vi "纳清pH_所有参数读取.vi"(8 "error in (no error)":errorcluster caption="错误输入（无错误）", 11 "MB session in":refnum<class "MB_Master.lvclass">) -> (0 "error out":errorcluster caption="错误输出", 2 "输出值":T1 {"波特率" items=["4800", "9600", "19200", "38400", "57600", "115200"]}, 3 "MB session out":refnum<class "MB_Master.lvclass">)   [LabVIEW 2016, in "斯坦道多参数.lvlib"]
uses:
  <vilib>/Plasmionique/MB Master/MB_Master/MB_Master.lvclass
  <vilib>/Plasmionique/MB Master/MB Master.lvlib
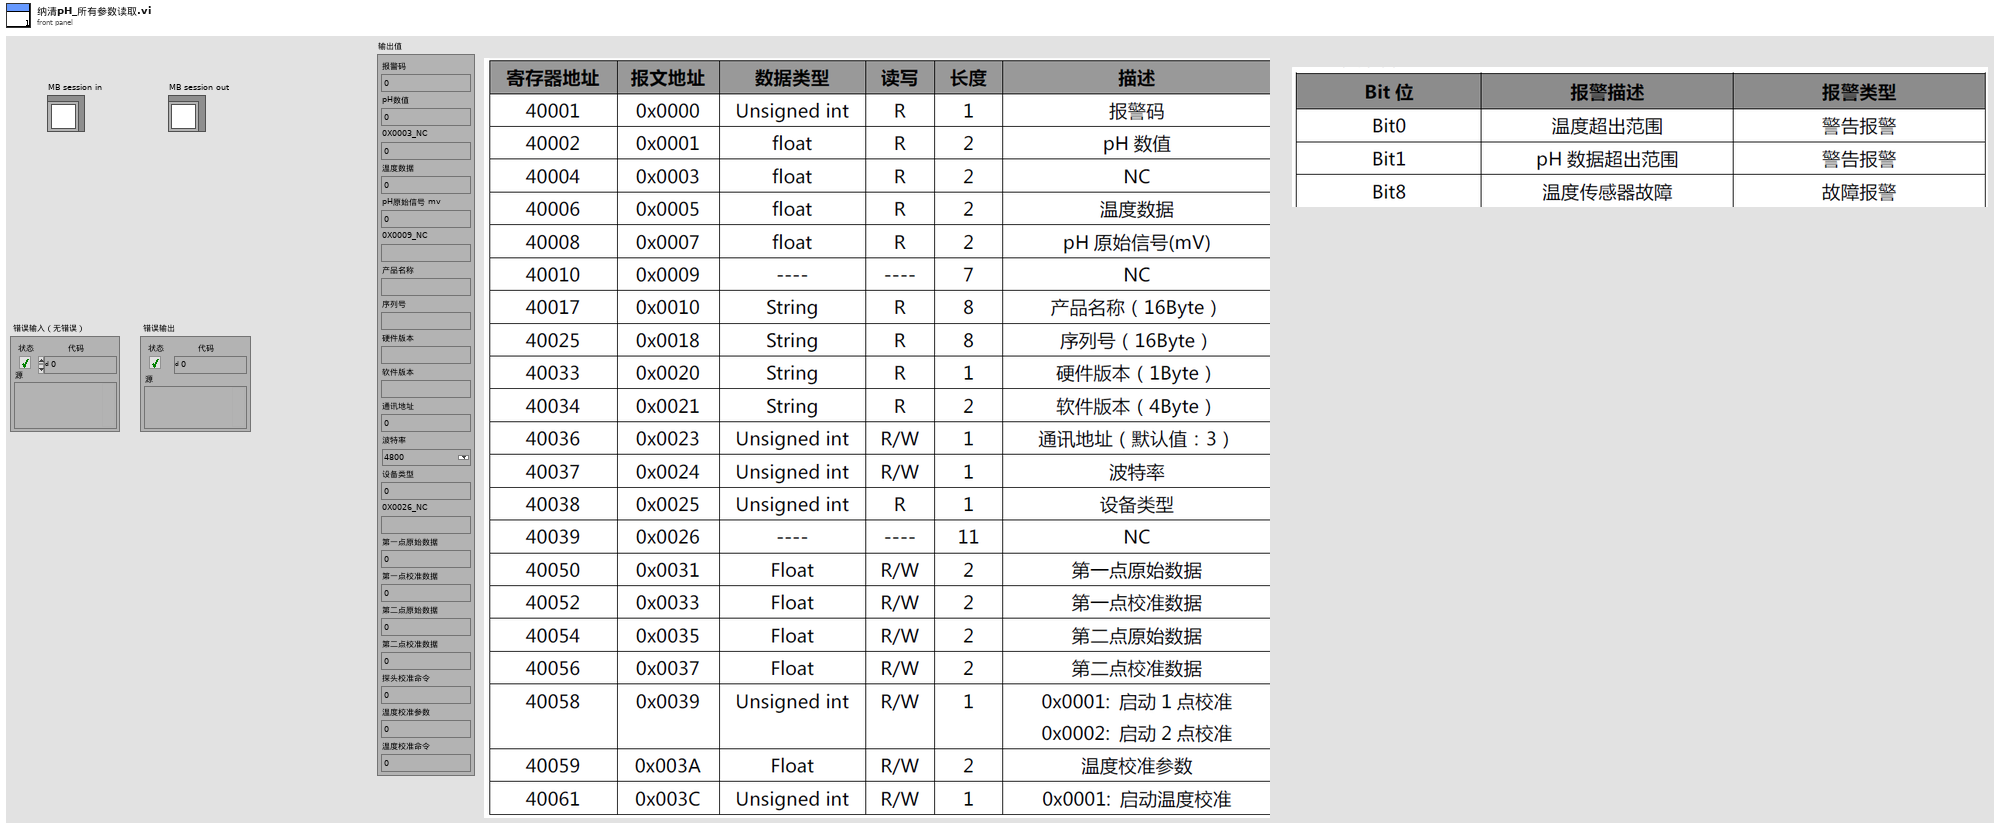
[diagram p1: front panel]
types:
  T1 = cluster{"报警码":u16, "pH数值":sgl, "0X0003_NC":sgl, "温度数据":sgl, "pH原始信号 mv":sgl, "0X0009_NC":string, "产品名称":string, "序列号":string, "硬件版本":string, "软件版本":string, "通讯地址":u16, "波特率":u16, "设备类型":u16, "0X0026_NC":string, "第一点原始数据":sgl, "第一点校准数据":sgl, "第二点原始数据":sgl, "第二点校准数据":sgl, "探头校准命令":u16, "温度校准参数":sgl, "温度校准命令":u16}
  T2 = cluster{"pH":u32, "DO":u32, "Cond":u32, "Turb":u32, "叶绿素a":u32, "藻密度":u32, "ORP":u32}
  T3 = cluster{u16, "mode":dbl, "数值":sgl, "数值":sgl, "数值":sgl, "类型":string, "类型":string, "类型":string, "类型":string, "类型":string, u16, u16, u16, "类型":string, "数值":sgl, "数值":sgl, "数值":sgl, "数值":sgl, u16, "数值":sgl, u16}
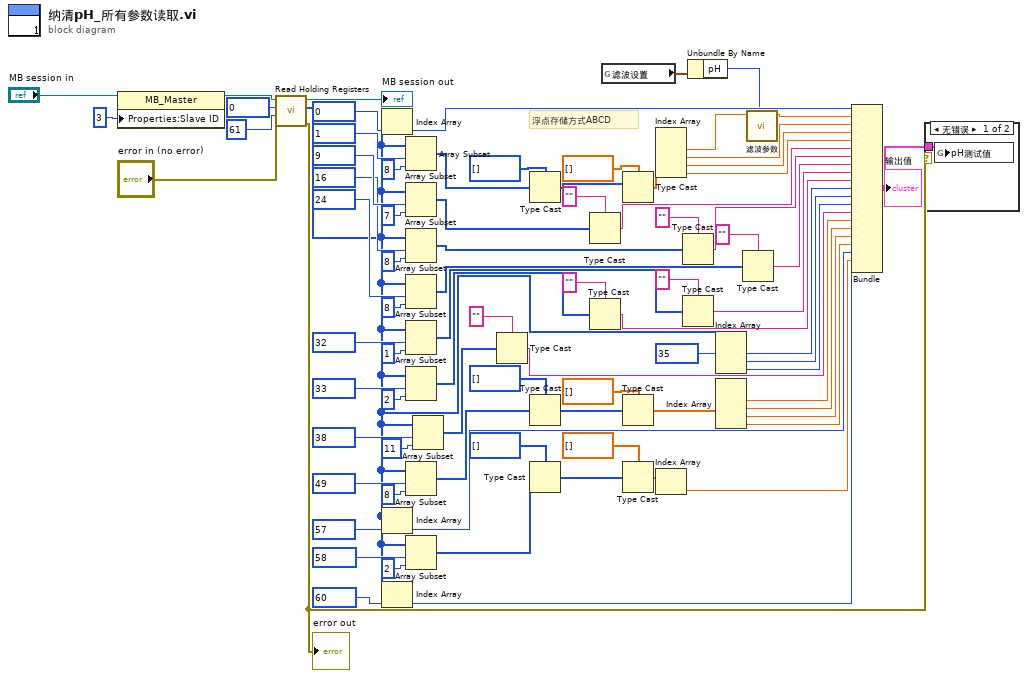
[diagram p0: block diagram]
diagram:
  # "浮点存储方式ABCD"
  n1 = property class="MB_Master"(reference="MB session in", "Properties:Slave ID"=u8 3 ("Slave ID")) -> (reference out=w73:refnum<class "MB_Master.lvclass">)  [unwired: 1 in, 1 out]
  n2 = call <vilib>:"Read Holding Registers.vi"("error in (no error)"="error in (no error)", "quantity"=u16 61, "starting address"=u16 0, "MB session in"=w73) -> ("error out"=w14:errorcluster, "Registers"=w16:u16[], "MB session out"=→"MB session out":refnum<class "MB_Master.lvclass">)  [unwired: 5 in]
  "error out" <- w14
  n3 = Index Array(array=w16, index=u16 0 ("starting address")) -> (element=w81:u16)
  n4 = Index Array(array=w16, index=u16 57 ("starting address")) -> (element=w19:u16)
  n5 = Index Array(array=w16, index=u16 60 ("starting address")) -> (element=w15:u16)
  n6 = Array Subset(array=w16, index=u16 1 ("starting address"), length=8 ("长度")) -> (w77:u16[])
  n7 = Array Subset(array=w16, index=u16 9 ("starting address"), length=7 ("长度")) -> (w67:u16[])
  n8 = Array Subset(array=w16, index=u16 16 ("starting address"), length=8 ("长度")) -> (w63:u16[])
  n9 = Array Subset(array=w16, index=u16 24 ("starting address"), length=8 ("长度")) -> (w57:u16[])
  n10 = Array Subset(array=w16, index=u16 32 ("starting address"), length=1 ("长度")) -> (w53:u16[])
  n11 = Array Subset(array=w16, index=u16 33 ("starting address"), length=2 ("长度")) -> (w47:u16[])
  n12 = Array Subset(array=w16, index=u16 49 ("starting address"), length=8 ("长度")) -> (w34:u16[])
  n13 = Array Subset(array=w16, index=u16 58 ("starting address"), length=2 ("长度")) -> (w22:u16[])
  n14 = Array Subset(array=w16, index=u16 38 ("starting address"), length=11 ("长度")) -> (w37:u16[])
  n15 = Type Cast(type="" ("类型"), x=w37) -> (*(type *) &x=w36:string)
  n16 = Type Cast(type=u32[] [] ("数组 2"), x=w77) -> (*(type *) &x=w13:u32[])
  n17 = Type Cast(type=u32[] [] ("数组 2"), x=w34) -> (*(type *) &x=w32:u32[])
  n18 = Type Cast(type=u32[] [] ("数组 2"), x=w22) -> (*(type *) &x=w24:u32[])
  n19 = Type Cast(type="" ("类型"), x=w67) -> (*(type *) &x=w65:string)
  n20 = Type Cast(type="" ("类型"), x=w47) -> (*(type *) &x=w45:string)
  n21 = global read "断电保存变量.vi" "滤波设置"() -> (w2:T2)
  n22 = Type Cast(type=sgl[] [] ("数组 2"), x=w13) -> (*(type *) &x=w76:sgl[])
  n23 = Type Cast(type=sgl[] [] ("数组 2"), x=w32) -> (*(type *) &x=w29:sgl[])
  n24 = Type Cast(type=sgl[] [] ("数组 2"), x=w24) -> (*(type *) &x=w27:sgl[])
  n25 = Index Array(array=w76) -> (element #1=w4:sgl, element #2=w71:sgl, element #3=w10:sgl, element #4=w9:sgl)  [unwired: 4 in]
  n26 = Index Array(array=w27) -> (element=w18:sgl)  [unwired: 1 in]
  n27 = Type Cast(type="" ("类型"), x=w63) -> (*(type *) &x=w60:string)
  n28 = Type Cast(type="" ("类型"), x=w53) -> (*(type *) &x=w50:string)
  n29 = Unbundle By Name(w2) -> ("pH"=w1:u32)
  n30 = Index Array(array=w16, index #1=u16 35 ("starting address")) -> (element #1=w43:u16, element #2=w42:u16, element #3=w41:u16)  [unwired: 2 in]
  n31 = Index Array(array=w29) -> (element #1=w28:sgl, element #2=w8:sgl, element #3=w7:sgl, element #4=w6:sgl)  [unwired: 4 in]
  n32 = Type Cast(type="" ("类型"), x=w57) -> (*(type *) &x=w55:string)
  n33 = call "滤波参数.vi"("滤波次数"=w1, "x"=w4) -> ("mode"=w3:dbl)  [unwired: 9 in]
  n34 = Bundle(w81, "mode"=w3, "数值"=w71, "数值"=w10, "数值"=w9, "类型"=w65, "类型"=w60, "类型"=w55, "类型"=w50, "类型"=w45, w43, w42, w41, "类型"=w36, "数值"=w28, "数值"=w8, "数值"=w7, "数值"=w6, w19, "数值"=w18, w15) -> (w5:T3)  [unwired: 1 in]
  "输出值" <- w5
  n35 = case shown="无错误" w14 {
    tunnel: w5 -> [w84 _]
    frame No Error {
      n36 = global write "纳清过程全局变量.vi" "pH测试值"(w84) -> ()
    }
    frame Error {
    }
  }
